vi "LaunchNewProjectDialog.vi"   [LabVIEW 2016]
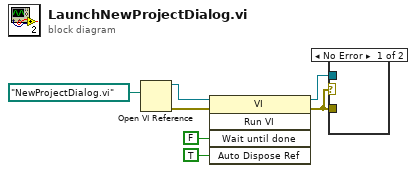
[diagram p0: block diagram]
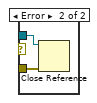
[diagram p2: hidden frame]
diagram:
  n1 = Open VI Reference(vi path=path "NewProjectDialog.vi") -> (vi reference=w5:refnum<vi>, error out=w4:errorcluster)  [unwired: 5 in]
  n2 = invoke class="VI" method="Run VI"(reference=w5, error in=w4, "Wait until done"=FALSE ("Wait Until Done"), "Auto Dispose Ref"=TRUE ("Auto Dispose Reference")) -> (reference out=w3:refnum<vi>, error out=w2:errorcluster)  [unwired: 1 in, 3 out]
  n3 = case shown="No Error" w2 {
    tunnel: w3 -> [_ w9]
    tunnel: w2 -> [_ w8]
    frame No Error {
    }
    frame Error {
      n4 = Close Reference(reference=w9, error in (no error)=w8) -> ()  [unwired: 1 out]
    }
  }
